vi "FFT - APS MAG+Phase (NOT implemented).vi"(0 "reference in":refnum<class "GSwFormDSP.lvclass">, 5 "error in (no error)":errorcluster) -> (13 "Nb Averages":i32[](array[numeric]), 14 "reference out":refnum<class "GSwFormDSP.lvclass">, 19 "error out":errorcluster)   [LabVIEW 2022 SP3, in "GSwFormDSP.lvclass"]
uses:
  GSwFormDSP.lvclass
  <vilib>/Analysis/0measdsp.llb/Scaled Time Domain Window (DBL).vi
  <vilib>/Analysis/NI_AALPro.lvlib
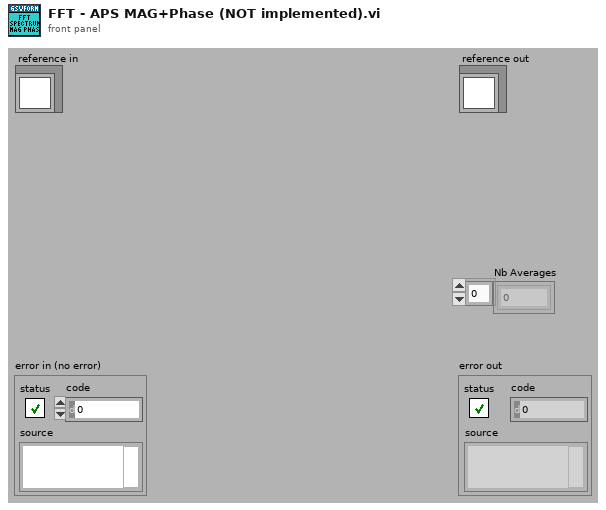
[diagram p1: front panel]
types:
  T1 = typedef "GSwFormDSP.lvclass/ObjectAttributesRef.ctl" = refnum<data-value>
  T2 = typedef "GSwFormDSP.lvclass/ObjectAttributes.ctl" = cluster{"Wform Ref":refnum<data-value>, "Nb Signals":i32, "Spectral Function Parameters":T3, "FFT":waveform(cdb)[], "Nb FFT":i32, "Nb Averages":i32[], "Reference Indexes":i32[], "Response Indexes":i32[], "Coherence":waveform(dbl)[], "TDF Parameters":T5, "DAQ":cluster{"Duration (sec)":dbl, "Buffer Size (Samples)":i32, "Offset (Samples)":i32}, "Filter Impulse Response (TDF)":waveform(dbl), "Sound Playback":T6}
  T3 = typedef "GSwFormDSP.lvclass/Spectral Parameters.ctl" = cluster{"Frequency resolution (Hz)":dbl, "Overlap":dbl, "Window":T4}
  T4 = typedef "NI_AALPro.lvlib/windowTd.ctl" = u32
  T5 = typedef "GSwFormDSP.lvclass/TDF Parameters.ctl" = cluster{"Filter":enum32{"Lowpass", "Highpass", "Bandpass", "Bandstop"}, "Type:":enum16{"Butterworth", "Chebyshev", "Inv Chebyshev", "Elliptic", "Bessel"}, "LP cutoff freq":dbl, "HP cutoff freq":dbl, "Order":i32, "passband ripple (dB)":dbl, "stopband attenuation (dB)":dbl, "Phaseless Filter":bool, "Include Fade IN and OUT":bool}
  T6 = typedef "GSwFormDSP.lvclass/Sound Playback.ctl" = cluster{"Timer start (ms)":u32, "task ID":T7, "Cursor Init Location (s)":dbl, "SC Volume":dbl}
  T7 = typedef "Sound Output Task ID.ctl" = u32
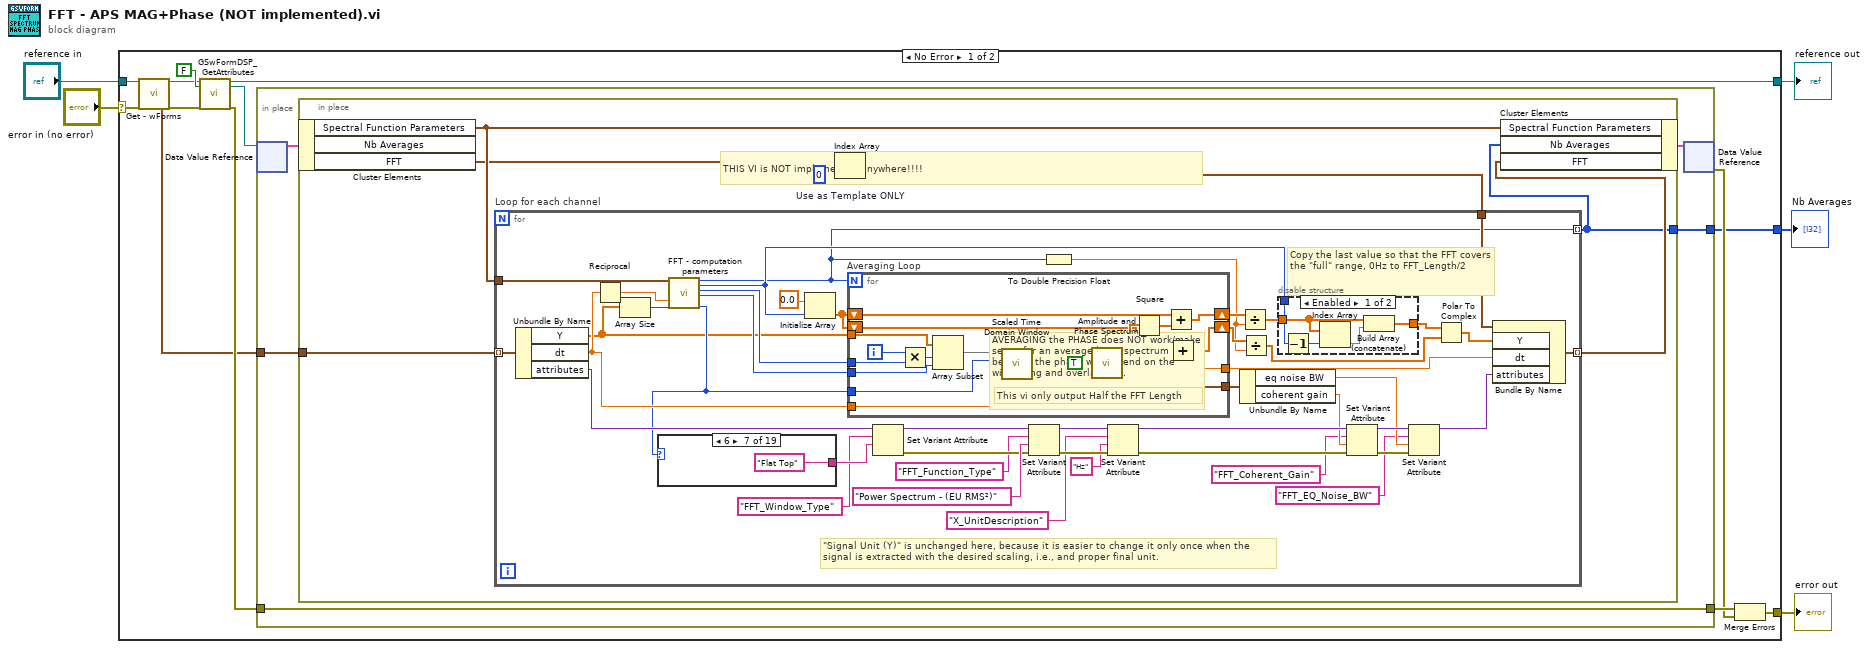
[diagram p0: block diagram]
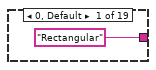
[diagram p3: hidden frame]
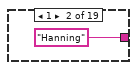
[diagram p4: hidden frame]
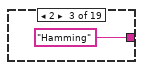
[diagram p5: hidden frame]
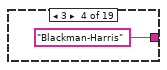
[diagram p6: hidden frame]
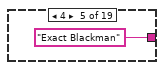
[diagram p7: hidden frame]
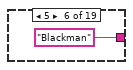
[diagram p8: hidden frame]
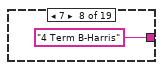
[diagram p9: hidden frame]
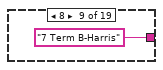
[diagram p10: hidden frame]
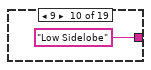
[diagram p11: hidden frame]
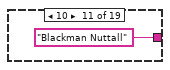
[diagram p12: hidden frame]
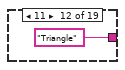
[diagram p13: hidden frame]
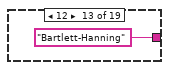
[diagram p14: hidden frame]
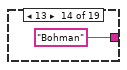
[diagram p15: hidden frame]
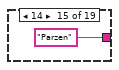
[diagram p16: hidden frame]
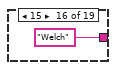
[diagram p17: hidden frame]
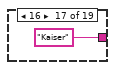
[diagram p18: hidden frame]
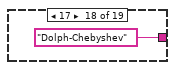
[diagram p19: hidden frame]
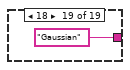
[diagram p20: hidden frame]
diagram:
  n1 = case shown="No Error" "error in (no error)" {
    selector: "error in (no error)" -> [w9 w121]
    tunnel: [w18 w121] -> w4
    tunnel: [w14 w120] -> w2
    tunnel: "reference in" -> [w10 w120]
    tunnel: [w11 i32[] []] -> w1
    frame No Error {
      n2 = call-dynamic "Get - wForms.vi"("reference in"=w10, "error in (no error)"=w9) -> ("wForms"=w6:waveform(dbl)[], "reference out"=w7:refnum<class "GSwFormDSP.lvclass">, "error out"=w8:errorcluster)  [unwired: 14 in, 1 out]
      n3 = call "GSwFormDSP_GetAttributes.vi"("reference in"=w7, "return data? (T)"=FALSE, "error in (no error)"=w8) -> ("reference out"=w14:refnum<class "GSwFormDSP.lvclass">, "attributes ref"=w13:T1, "error out"=w15:errorcluster)  [unwired: 13 in, 1 out]
      n4 = in-place {
        in-place-border: w15 -> [w21]
        in-place-border: [w21] -> w17
        in-place-border: [w20] -> w11
        in-place-border: w6 -> [w19]
        n5 = in-place-dvr #1(w13) -> (w22:T2)  [unwired: 1 out]
        n6 = in-place {
          in-place-border: [w25] -> w20
          in-place-border: w19 -> [w24]
          # "THIS VI is NOT implemented anywhere!!!!"
          n7 = in-place-cluster #2(w22) -> ("Spectral Function Parameters"=w29:T3, "FFT"=w28:waveform(cdb)[])  [unwired: 1 out]
          n8 = Index Array "Use as Template ONLY"(array=w28, index=0) -> (element=w26:waveform(cdb))
          n9 = for "Loop for each channel" {
            tunnel: w24 -> [w38] mode=indexing
            tunnel: [w74] -> w30 mode=indexing
            tunnel: w29 -> [w73]
            tunnel: w26 -> [w40]
            tunnel: [w37] -> w25 mode=indexing
            # "Copy the last value so that the FFT covers the \"full\" range, 0Hz to FFT_Length/2"
            # "\"Signal Unit (Y)\" is unchanged here, because it is easier to change it only once when the signal is extracted with the desired scaling, i.e., and proper final unit."
            n10 = Unbundle By Name(w38) -> ("Y"=w39:dbl[], "dt"=w66:dbl, "attributes"=w65:variant)
            n11 = Reciprocal(x=w66) -> (1/x=w67:dbl)
            n12 = Array Size(array=w39) -> (size(s)=w68:i32)
            n13 = call "FFT - computation parameters.vi"("Spectral Function Parameters"=w73, "Fs"=w67, "Time vector length (samples)"=w68) -> ("Nb Averages"=w37:i32, "FFT Length/2"=w42:i32, "FFT Length - Overlap"=w69:i32, "FFT Length"=w44:i32, "window"=w41:T4)  [unwired: 11 in, 1 out]
            n14 = case shown="6" w41 {
              tunnel: ["Rectangular" ("Abscissa.Unit (X)") "Hanning" ("Abscissa.Unit (X)") "Hamming" ("Abscissa.Unit (X)") "Blackman-Harris" ("Abscissa.Unit (X)") "Exact Blackman" ("Abscissa.Unit (X)") "Blackman" ("Abscissa.Unit (X)") "Flat Top" ("Abscissa.Unit (X)") "4 Term B-Harris" ("Abscissa.Unit (X)") "7 Term B-Harris" ("Abscissa.Unit (X)") "Low Sidelobe" ("Abscissa.Unit (X)") "Blackman Nuttall" ("Abscissa.Unit (X)") "Triangle" ("Abscissa.Unit (X)") "Bartlett-Hanning" ("Abscissa.Unit (X)") "Bohman" ("Abscissa.Unit (X)") "Parzen" ("Abscissa.Unit (X)") "Welch" ("Abscissa.Unit (X)") "Kaiser" ("Abscissa.Unit (X)") "Dolph-Chebyshev" ("Abscissa.Unit (X)") "Gaussian" ("Abscissa.Unit (X)")] -> w63
              frame 0, Default {
              }
              frame 1 {
              }
              frame 2 {
              }
              frame 3 {
              }
              frame 4 {
              }
              frame 5 {
              }
              frame 6 {
              }
              frame 7 {
              }
              frame 8 {
              }
              frame 9 {
              }
              frame 10 {
              }
              frame 11 {
              }
              frame 12 {
              }
              frame 13 {
              }
              frame 14 {
              }
              frame 15 {
              }
              frame 16 {
              }
              frame 17 {
              }
              frame 18 {
              }
            }
            n15 = Initialize Array(0.0, w42) -> (w36:dbl[])
            n16 = for "Averaging Loop" {
              N: w37 -> [_]
              shift-right: [w109] -> w71
              shift-left: w36 -> [w111]
              tunnel: w69 -> [w115]
              tunnel: w44 -> [w114]
              tunnel: w39 -> [w113]
              tunnel: w66 -> [w110]
              tunnel: [w108] -> w64
              tunnel: [w107] -> w70
              tunnel: w41 -> [w106]
              shift-right: [w100] -> w35
              shift-left: w36 -> [w102]
              i -> [w116]
              # "AVERAGING the PHASE does NOT work/make sense for an averaged autospectrum because the phase will depend on the windowing and overlap, etc."
              # "This vi only output Half the FFT Length"
              n17 = Multiply(x=w116, y=w115) -> (x*y=w117:i32)
              n18 = Array Subset(array=w113, index=w117, length=w114) -> (w112:dbl[])
              n19 = call-poly <vilib>:"Scaled Time Domain Window.vi"("window"=w106, "X"=w112) -> ("window properties"=w107:cluster{"eq noise BW":dbl, "coherent gain":dbl}, "Windowed X"=w118:dbl[])  [unwired: 1 in, 7 out]
              n20 = call <vilib>:"Amplitude and Phase Spectrum.vi"("dt"=w110, "unwrap phase (T)"=TRUE, "Signal (V)"=w118) -> ("df"=w108:dbl, "Amp Spectrum Phase (radians)"=w101:dbl[], "Amp Spectrum Mag (Vrms)"=w104:dbl[])
              n21 = Square(x=w104) -> (x^2=w103:dbl[])
              n22 = Add(x=w111, y=w103) -> (x+y=w109:dbl[])
              n23 = Add(x=w102, y=w101) -> (x+y=w100:dbl[])
            }
            n24 = Set Variant Attribute(Variant=w65, name="FFT_Window_Type" ("Att - Window Type"), value=w63) -> (Variant out=w62:variant, error out=w60:errorcluster)  [unwired: 1 in, 1 out]
            n25 = Set Variant Attribute(Variant=w62, name="FFT_Function_Type" ("Att - Function Type"), value="Power Spectrum - (EU RMS²)" ("Ordinate.Function Description.Function Type"), error in=w60) -> (Variant out=w59:variant, error out=w58:errorcluster)  [unwired: 1 out]
            n26 = To Double Precision Float(number=w37) -> (double precision float=w34:dbl)
            n27 = Set Variant Attribute(Variant=w59, name="X_UnitDescription" ("X unit"), value="Hz" ("Abscissa.Unit (X)"), error in=w58) -> (Variant out=w56:variant, error out=w55:errorcluster)  [unwired: 1 out]
            n28 = Divide(x=w71, y=w34) -> (x/y=w43:dbl[])
            n29 = Unbundle By Name(w70) -> ("eq noise BW"=w51:dbl, "coherent gain"=w54:dbl)
            n30 = Divide(x=w35, y=w34) -> (x/y=w31:dbl[])
            n31 = disable-structure shown="Enabled" {
              disable-tunnel: [w78 w80] -> w33
              disable-tunnel: w43 -> [w77 w80]
              disable-tunnel: w42 -> [w76 _]
              frame Enabled {
                n32 = Decrement(x=w76) -> (x-1=w75:i32)
                n33 = Index Array(array=w77, index=w75) -> (element=w79:dbl)
                n34 = Build Array (concatenate)(w77, w79) -> (w78:dbl[])
              }
              frame Disabled {
              }
            }
            n35 = Set Variant Attribute(Variant=w56, name="FFT_Coherent_Gain" ("Coherent Gain (DBL)"), value=w54, error in=w55) -> (Variant out=w52:variant, error out=w53:errorcluster)  [unwired: 1 out]
            n36 = Set Variant Attribute(Variant=w52, name="FFT_EQ_Noise_BW" ("EQ noise BW (DBL)"), value=w51, error in=w53) -> (Variant out=w50:variant)  [unwired: 2 out]
            n37 = Polar To Complex(1:w31, 2:w33) -> (0:w32:cdb[])
            n38 = Bundle By Name(cluster=w40, "Y"=w32, "dt"=w64, "attributes"=w50) -> (w74:waveform(cdb))
          }
          n39 = in-place-cluster #2("Spectral Function Parameters"=w29, "Nb Averages"=w25, "FFT"=w30) -> (w23:T2)
        }
        n40 = in-place-dvr #1(w23) -> (w12:errorcluster)  [unwired: 1 out]
      }
      n41 = Merge Errors(w17, w12) -> (w18:errorcluster)
    }
    frame Error {
    }
  }
  "error out" <- w4
  "reference out" <- w2
  "Nb Averages" <- w1
